vi "Acquire Waveform.vi"(8 "error in (no error)":errorcluster, 10 "Channel":i32(ring) items=["Channel 1"=0, "Channel 2"=1, "Channel 3"=2, "Channel 4"=3, "Waveform Memory 1"=5, "Waveform Memory 2"=6, "Serial Bus 1"=7, "Serial Bus 2"=8, "Digital Bus Low"=9, "Digital Bus High "=10, "Digital Bus 1"=11, "Digital Bus 2"=12, "External"=29, "Function 1"=32, "Function 2"=33, "Function 3"=34, "Function 4"=35, "Math 1"=36, "Math 2"=37, "Math 3"=38, "Math 4"=39, "FFT"=40, "Analog Bus"=41], 11 "Agilent 3054A in":refnum<class "Agilent 3054A.lvclass">) -> (0 "error out":errorcluster, 2 "Waveform Data":waveform(dbl)(graph), 3 "Agilent 3054A out":refnum<class "Agilent 3054A.lvclass">)   [LabVIEW 2016, in "Oscilloscope.lvlib" / "Agilent 3054A.lvclass"]
uses:
  Agilent 3054A.lvclass
  Agilent 3054A.lvclass/Agilent 3054A.ctl
  <instrlib>/Agilent 2000 3000 X-Series/Public/Data/Read Waveforms (Single).vi
  <instrlib>/Agilent 2000 3000 X-Series/Agilent 2000 3000 X-Series.lvlib
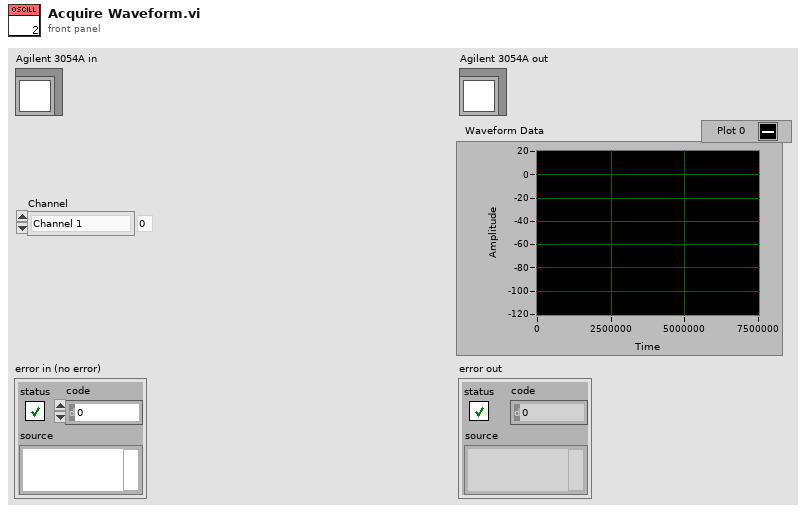
[diagram p1: front panel]
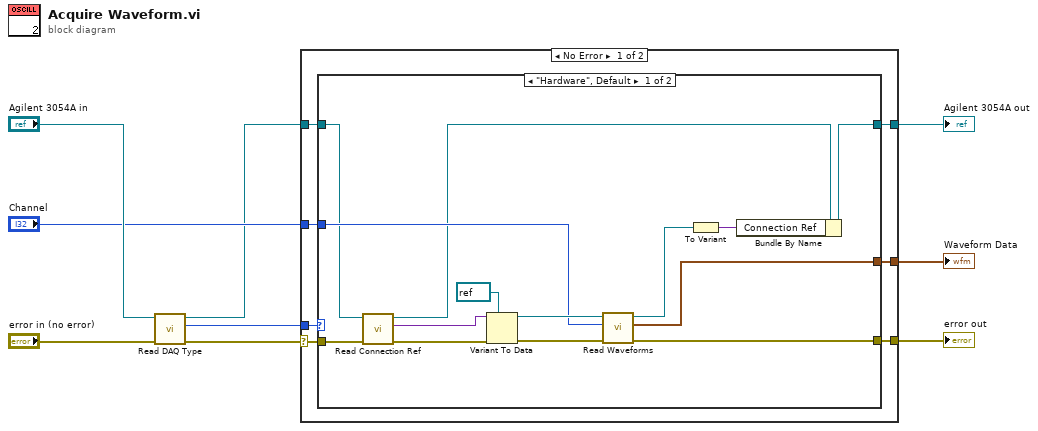
[diagram p0: block diagram]
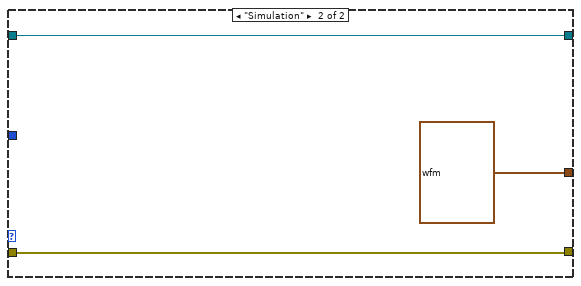
[diagram p2: hidden frame]
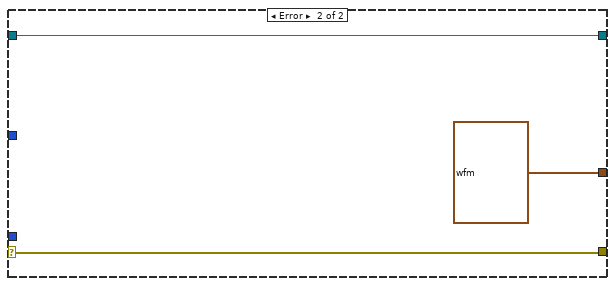
[diagram p3: hidden frame]
diagram:
  n1 = call-dynamic "Read DAQ Type.vi"("error in (no error)"="error in (no error)", "Agilent 3054A in"="Agilent 3054A in") -> ("error out"=w8:errorcluster, "DAQ Type"=w7:enum16{"Hardware", "Simulation"}, "Agilent 3054A out"=w1:refnum<class "Agilent 3054A.lvclass">)  [unwired: 7 in]
  n2 = case shown="No Error" w8 {
    selector: w8 -> [w14 w35]
    tunnel: w7 -> [w16 _]
    tunnel: w1 -> [w15 w36]
    tunnel: [w13 w36] -> w5
    tunnel: [w12 w35] -> w4
    tunnel: "Channel" -> [w11 _]
    tunnel: [w10 waveform(dbl) {"t0"=timestamp(0 s since 1904-01-01), "dt"=1.0, "Y"=[0.0]} ("Waveform Data")] -> w2
    frame No Error {
      n3 = case shown="\"Hardware\", Default" w16 {
        tunnel: w15 -> [w18 w33]
        tunnel: w14 -> [w30 w32]
        tunnel: [w24 w33] -> w13
        tunnel: [w25 w32] -> w12
        tunnel: w11 -> [w21 _]
        tunnel: [w20 waveform(dbl) {"t0"=timestamp(0 s since 1904-01-01), "dt"=1.0, "Y"=[0.0]} ("Waveform Data")] -> w10
        frame "Hardware", Default {
          n4 = call-dynamic "Read Connection Ref.vi"("error in (no error)"=w30, "Agilent 3054A in"=w18) -> ("error out"=w29:errorcluster, "Connection Ref"=w27:variant, "Agilent 3054A out"=w17:refnum<class "Agilent 3054A.lvclass">)  [unwired: 7 in]
          n5 = Variant To Data(error in=w29, type=refnum<visa-resource-name> refnum ("VISA resource name"), Variant=w27) -> (data=w22:refnum<visa-resource-name>, error out=w26:errorcluster)
          n6 = call-poly <instrlib>:"Read Waveforms.vi"("error in (no error)"=w26, "Source Channel (0: Channel 1)"=w21, "VISA resource name"=w22) -> ("error out"=w25:errorcluster, "Waveform Data"=w20:waveform(dbl), "VISA resource name out"=w23:refnum<visa-resource-name>)  [unwired: 6 in]
          n7 = To Variant(anything=w23) -> (Variant=w19:variant)
          n8 = Bundle By Name(cluster=w17, "Connection Ref"=w19) -> (w24:refnum<class "Agilent 3054A.lvclass">)
        }
        frame "Simulation" {
        }
      }
    }
    frame Error {
    }
  }
  "error out" <- w4
  "Agilent 3054A out" <- w5
  "Waveform Data" <- w2
